vi "PV ActiveLine - Display Resolution (TPG362).vi"(7 "W/R":bool, 8 "Fehler (Eingang)":errorcluster, 9 "Display control digits CH2":i32(ring) items=["Auto (default)", "One digit", "Two digits", "Three digits", "Four digits"], 10 "Display control digits":i32(ring) items=["Auto (default)", "One digit", "Two digits", "Three digits", "Four digits"], 11 "Referenz in":refnum<visa-resource-name>) -> (0 "Cluster (Ausgang)":errorcluster, 1 "Get Display control digits CH2":i32(ring) items=["Auto (default)", "One digit", "Two digits", "Three digits", "Four digits"], 2 "Get Display control digits":i32(ring) items=["Auto (default)", "One digit", "Two digits", "Three digits", "Four digits"], 3 "Referenz out":refnum<visa-resource-name>)   [LabVIEW 2013, in "PV ActiveLine.lvlib"]
doc: "DCD - Display Resolution\n\nTransmit: DCD [a,a]\nReceive: a,a\n\nResolution a =\n0 –> AUTO (default)\n1 –> One digit\n2 –> Two digits\n3 –> Three digits\n4 –> Four digits\n\nWhen the PrE is ON and the pressure is in the range p<1.0E-4 hPa the display resolution of the PCR Gauge is reduced by one decimal digit."
uses:
  <instrlib>/PV ActiveLine/PV ActiveLine.lvlib
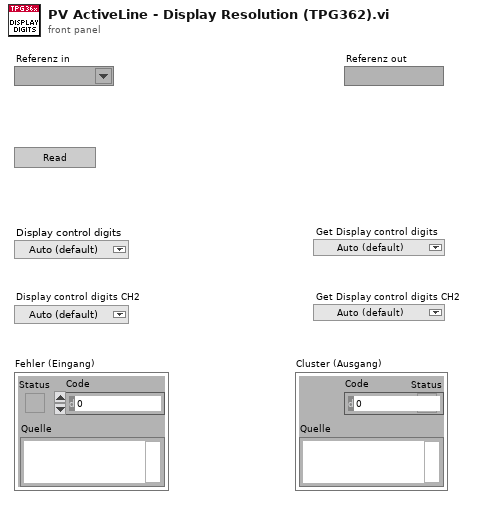
[diagram p1: front panel]
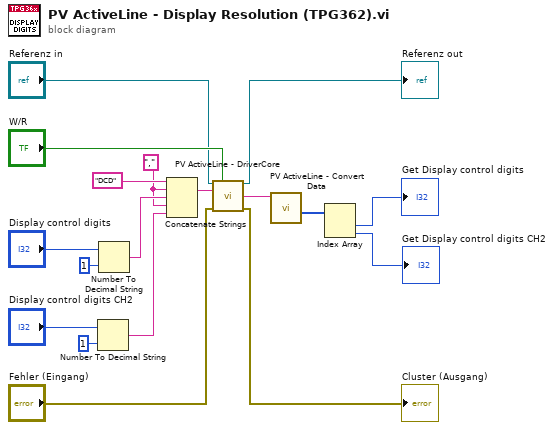
[diagram p0: block diagram]
diagram:
  w6 = "," ("Command")
  n1 = Number To Decimal String(number="Display control digits CH2", width (-)=i16 1) -> (decimal integer string=w5:string)
  n2 = Number To Decimal String(number="Display control digits", width (-)=i16 1) -> (decimal integer string=w16:string)
  n3 = Concatenate Strings("DCD" ("Command"), w6, w16, w6, w5) -> (w14:string)
  n4 = call <instrlib>:"PV ActiveLine - DriverCore.vi"("Referenz in"="Referenz in", "Write/Read"="W/R", "Command"=w14, "Fehler (Eingang)"="Fehler (Eingang)") -> ("Referenz out"=→"Referenz out":refnum<visa-resource-name>, "String Out"=w4:string, "Cluster (Ausgang)"=→"Cluster (Ausgang)":errorcluster)  [unwired: 9 in]
  n5 = call <instrlib>:"PV ActiveLine - Convert Data.vi"("String in"=w4) -> ("Integer Out"=w3:i32[])  [unwired: 7 in, 3 out]
  n6 = Index Array(array=w3) -> (element #1=→"Get Display control digits":i32, element #2=→"Get Display control digits CH2":i32)  [unwired: 2 in]
